vi "Position to XML.vi"(8 "error in (no error)":errorcluster, 11 "StageSPIM in":refnum<class "StageSPIM.lvclass">) -> (0 "error out":errorcluster, 2 "XML string":string, 3 "StageSPIM out":refnum<class "StageSPIM.lvclass">)   [LabVIEW 2012, in "StageSPIM.lvclass"]
uses:
  StageSPIM.lvclass
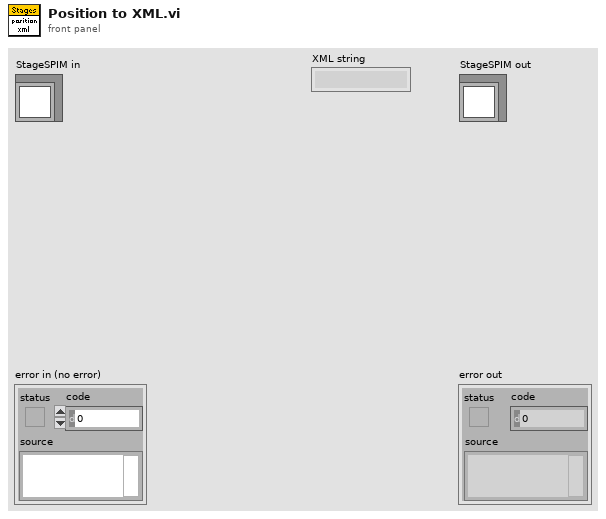
[diagram p1: front panel]
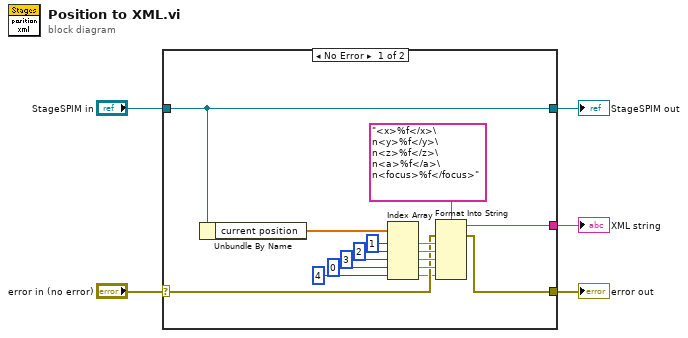
[diagram p0: block diagram]
diagram:
  n1 = case shown="No Error" "error in (no error)" {
    selector: "error in (no error)" -> [w10 w23]
    tunnel: [w9 w23] -> w4
    tunnel: [w21 w22] -> w2
    tunnel: "StageSPIM in" -> [w21 w22]
    tunnel: [w8 _] -> w1
    frame No Error {
      n2 = Unbundle By Name(w21) -> ("current position"=w20:dbl[])
      n3 = Index Array(array=w20, index #1=1 ("index"), index #2=2 ("index"), index #3=3 ("index"), index #4=0 ("index"), index #5=4 ("index")) -> (element #1=w14:dbl, element #2=w13:dbl, element #3=w12:dbl, element #4=w11:dbl, element #5=w6:dbl)
      n4 = Format Into String(format string="<x>%f</x>\n<y>%f</y>\n<z>%f</z>\n<a>%f</a>\n<focus>%f</focus>", error in=w10, w14, w13, w12, w11, w6) -> (resulting string=w8:string, error out=w9:errorcluster)  [unwired: 1 in]
    }
    frame Error {
    }
  }
  "error out" <- w4
  "StageSPIM out" <- w2
  "XML string" <- w1
